vi "Swap array elements 2D[Path].vi"(6 "Select":enum16{"Row", "Col"}(ring), 7 "Swap?":bool=TRUE, 9 "Index2":i32, 10 "Index1":i32, 11 "Input":path[][](array[path])) -> (3 "Output":path[][](array[path]))   [LabVIEW 2012]
doc: "功能：\n\n交换数组相邻两个元素的值，常见于数组冒泡排序中。\n\nSwap?1布尔输入端子用来选择交换数组的相邻元素，默认为FALSE，不交换。\n\nX[i+1]-->X[i]\n\nX[i]---->X[i+1]\n\ncsxcs_366创建"
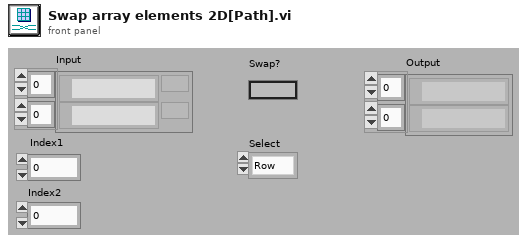
[diagram p1: front panel]
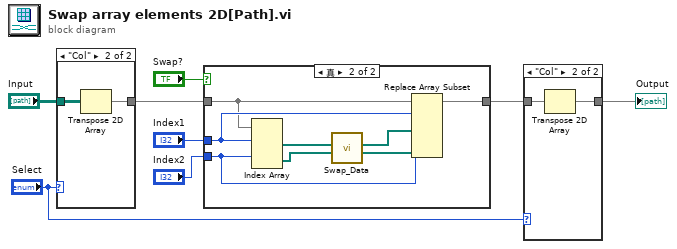
[diagram p0: block diagram]
diagram:
  n1 = case shown="\"Col\"" "Select" {
    tunnel: [w9 w11] -> w5
    tunnel: "Input" -> [w9 w10]
    frame "Row", Default {
    }
    frame "Col" {
      n2 = Transpose 2D Array(2D array=w10) -> (transposed array=w11:path[][])
    }
  }
  n3 = case shown="真" "Swap?" {
    tunnel: w5 -> [w12 w19]
    tunnel: [w12 w18] -> w2
    tunnel: "Index1" -> [_ w20]
    tunnel: "Index2" -> [_ w17]
    frame False {
    }
    frame True {
      n4 = Index Array(array=w19, index (row) #1=w20, index (row) #2=w17) -> (element #1=w16:path[], element #2=w15:path[])  [unwired: 2 in]
      n5 = call-poly "Swap_Data.vi"("b"=w15, "a"=w16) -> ("b"=w13:path[], "a"=w14:path[])  [unwired: 5 in]
      n6 = Replace Array Subset(array=w19, new element #1=w14, index (row) #1=w20, new element #2=w13, index (row) #2=w17) -> (w18:path[][])  [unwired: 2 in]
    }
  }
  n7 = case shown="\"Col\"" "Select" {
    tunnel: w2 -> [w21 w23]
    tunnel: [w21 w22] -> w1
    frame "Row", Default {
    }
    frame "Col" {
      n8 = Transpose 2D Array(2D array=w23) -> (transposed array=w22:path[][])
    }
  }
  "Output" <- w1
